vi "Config Heater Range.vi"(0 "VISA resource name":refnum<visa-resource-name>, 2 "Heater Range (0: Off)":u16(ring) items=["Off", "1", "2", "3", "4", "5"], 11 "error in (no error)":errorcluster) -> (4 "VISA resource name out":refnum<visa-resource-name>, 15 "error out":errorcluster)   [LabVIEW 2019, in "User lib.lvlib"]
doc: "This VI Configures the 340 Control Parameters, functions configured are PID, Heater Range, and Manual Output."
uses:
  SubVI/User lib.lvlib
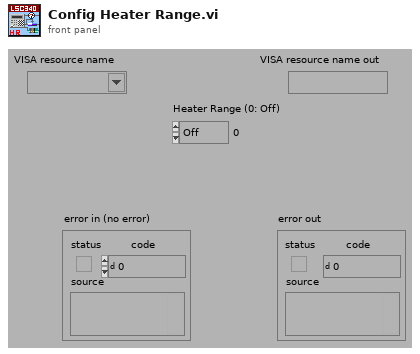
[diagram p1: front panel]
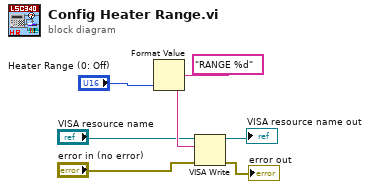
[diagram p0: block diagram]
diagram:
  n1 = Format Value(format string="RANGE %d", value (0)="Heater Range (0: Off)") -> (output string=w5:string)  [unwired: 1 in]
  n2 = VISA Write(VISA resource name="VISA resource name", write buffer=w5, error in (no error)="error in (no error)") -> (VISA resource name out=→"VISA resource name out":refnum<visa-resource-name>, error out=→"error out":errorcluster)  [unwired: 1 out]
